vi "XML.ControlToString.vi"(8 "error in":errorcluster, 11 "control ref in":refnum<vi>) -> (0 "error out":errorcluster, 1 "string value":string, 2 "label":string, 3 "control ref out":refnum<vi>)   [LabVIEW 2019, in "Tools.lvlib"]
uses:
  Tools.lvlib
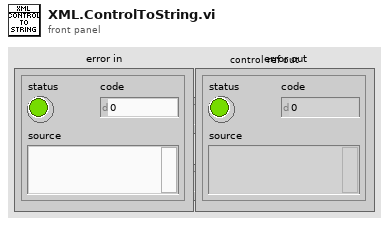
[diagram p1: front panel]
types:
  T1 = typedef "LVStringsAndValuesArrayTypeDef.ctl" = cluster{"String":string, "Value":ext}[]
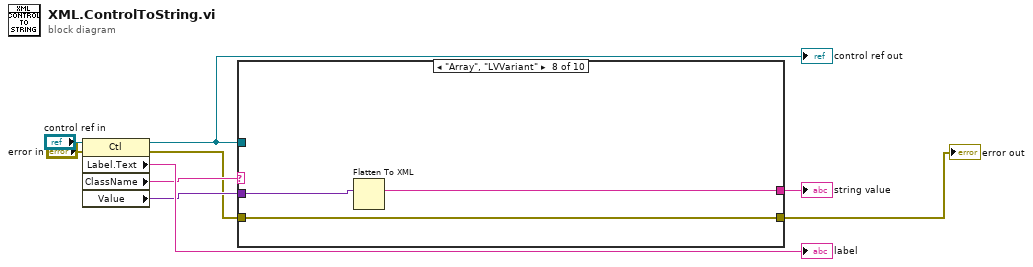
[diagram p0: block diagram]
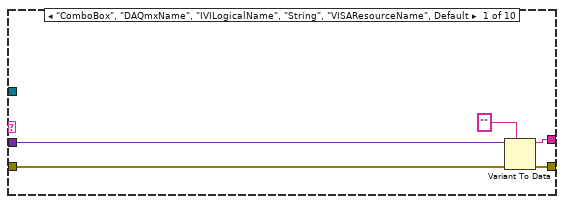
[diagram p2: hidden frame]
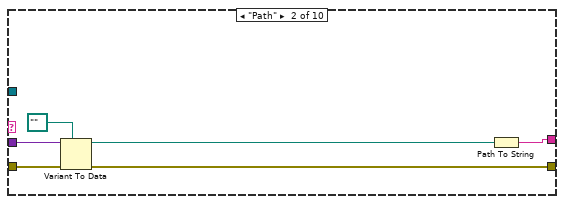
[diagram p3: hidden frame]
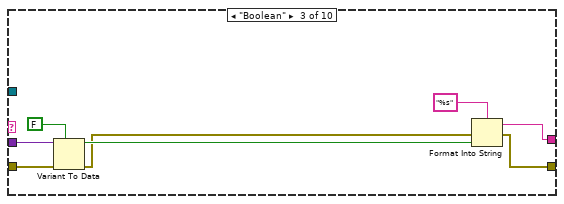
[diagram p4: hidden frame]
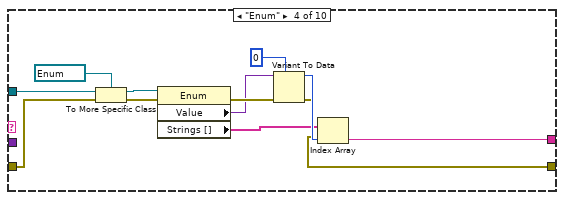
[diagram p5: hidden frame]
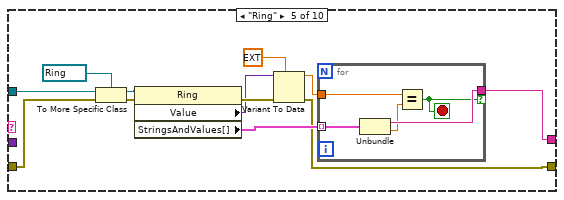
[diagram p6: hidden frame]
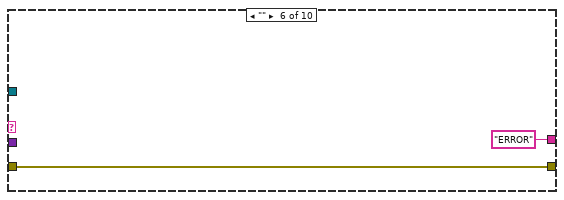
[diagram p7: hidden frame]
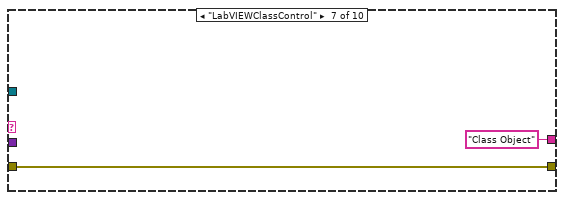
[diagram p8: hidden frame]
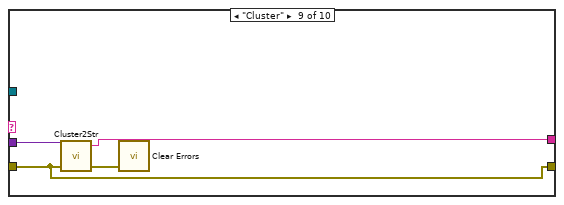
[diagram p9: hidden frame]
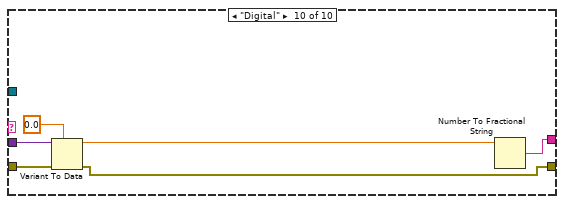
[diagram p10: hidden frame]
diagram:
  n1 = property class="Ctl"(reference="control ref in", error in="error in") -> (reference out=w8:refnum<vi>, error out=w2:errorcluster, "Label.Text"=→"label":string, "ClassName"=w5:string, "Value"=w6:variant)
  "control ref out" <- w8
  n2 = case shown="\"Array\", \"LVVariant\"" w5 {
    tunnel: w6 -> [w14 w18 w27 _ _ _ _ w63 w68 w73]
    tunnel: [w12 w17 w24 w31 w44 "ERROR" "Class Object" ("Formatted data out") w62 w67 w71] -> w7
    tunnel: w8 -> [_ _ _ w32 w46 _ _ _ _ _]
    tunnel: w2 -> [w11 w16 w23 w30 w42 w58 w61 w64 w66 w70]
    tunnel: [w10 w15 w21 w29 w41 w58 w61 w64 w66 w69] -> w1
    frame "ComboBox", "DAQmxName", "IVILogicalName", "String", "VISAResourceName", Default {
      n3 = Variant To Data(error in=w11, type="", Variant=w14) -> (data=w12:string, error out=w10:errorcluster)
    }
    frame "Path" {
      n4 = Variant To Data(error in=w16, type=path "", Variant=w18) -> (data=w19:path, error out=w15:errorcluster)
      n5 = Path To String(path=w19) -> (string=w17:string)
    }
    frame "Boolean" {
      n6 = Variant To Data(error in=w23, type=FALSE, Variant=w27) -> (data=w26:bool, error out=w22:errorcluster)
      n7 = Format Into String(format string="%s", error in=w22, w26) -> (resulting string=w24:string, error out=w21:errorcluster)  [unwired: 1 in]
    }
    frame "Enum" {
      n8 = To More Specific Class(target class=refnum<vi> refnum ("TESTITEM"), reference=w32, error in=w30) -> (specific class reference=w34:refnum<vi>, error out=w35:errorcluster)
      n9 = property class="Enum"(reference=w34, error in=w35) -> (error out=w40:errorcluster, "Value"=w37:variant, "Strings []"=w36:string[])  [unwired: 1 out]
      n10 = Variant To Data(error in=w40, type=0 ("Index"), Variant=w37) -> (data=w39:i32, error out=w29:errorcluster)
      n11 = Index Array(array=w36, index=w39) -> (element=w31:string)
    }
    frame "Ring" {
      n12 = To More Specific Class(target class=refnum<vi> refnum ("TESTITEM"), reference=w46, error in=w42) -> (specific class reference=w48:refnum<vi>, error out=w49:errorcluster)
      n13 = property class="Ring"(reference=w48, error in=w49) -> (error out=w52:errorcluster, "Value"=w50:variant, "StringsAndValues[]"=w45:T1)  [unwired: 1 out]
      n14 = Variant To Data(error in=w52, type=ext 0.0 ("Index"), Variant=w50) -> (data=w43:ext, error out=w41:errorcluster)
      n15 = for {
        tunnel: w45 -> [w57] mode=indexing
        tunnel: [w56] -> w44 if=w53
        tunnel: w43 -> [w54]
        stop <- w53 stop-if-true
        n16 = Unbundle(w57) -> ("String"=w56:string, "Value"=w55:ext)
        n17 = Equal?(x=w54, y=w55) -> (x = y?=w53:bool)
      }
    }
    frame "" {
    }
    frame "LabVIEWClassControl" {
    }
    frame "Array", "LVVariant" {
      n18 = Flatten To XML(anything=w63) -> (xml string=w62:string)
    }
    frame "Cluster" {
      n19 = call "Cluster2Str.vi"("error in (no error)"=w66, "Data_Cluster"=w68) -> ("error out"=w65:errorcluster, "Formatted data out"=w67:string)  [unwired: 2 in]
      n20 = call <vilib>:"Clear Errors.vi"("error in (no error)"=w65) -> ()  [unwired: 5 in, 2 out]
    }
    frame "Digital" {
      n21 = Variant To Data(error in=w70, type=0.0, Variant=w73) -> (data=w72:dbl, error out=w69:errorcluster)
      n22 = Number To Fractional String(number=w72) -> (F-format string=w71:string)  [unwired: 3 in]
    }
  }
  "string value" <- w7
  "error out" <- w1
